vi "Flatten Value.vi"(8 "error in (no error)":errorcluster, 11 "Boolean in":refnum<class "Test Executive 1D.lvclass">) -> (0 "error out":errorcluster, 2 "Value":string, 3 "Boolean out":refnum<class "Test Executive 1D.lvclass">)   [LabVIEW 2017, in "Custom Type Test Executive.lvlib" / "Test Executive 1D.lvclass"]
uses:
  <vilib>/gpm_packages/@cs/test-executive/Source/Custom Type Test Executive/Test Executive 1D Data Type/Test Executive 1D.lvclass
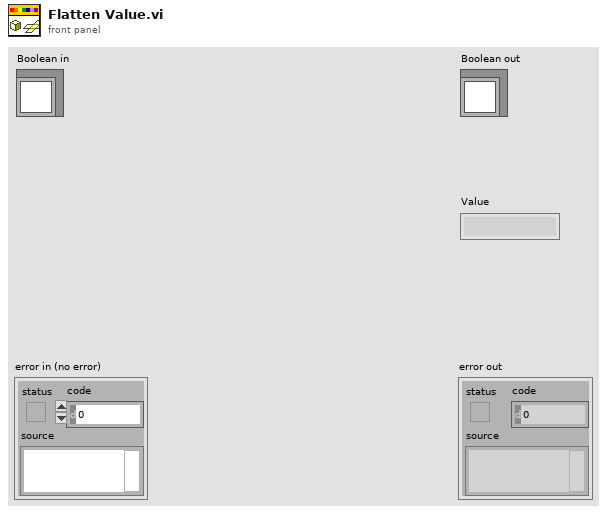
[diagram p1: front panel]
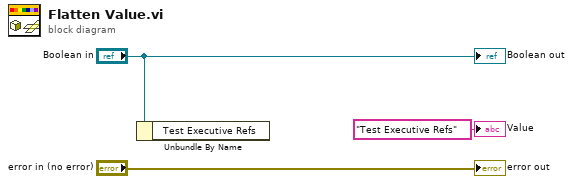
[diagram p0: block diagram]
diagram:
  n1 = Unbundle By Name("Boolean in") -> ()  [unwired: 1 out]
  "error out" <- "error in (no error)"
  "Boolean out" <- "Boolean in"
  "Value" <- "Test Executive Refs" ("Value")
